vi "Create Message.vi"(8 "error in (no error)":errorcluster, 11 "Message Name":string) -> (0 "error out":errorcluster, 3 "Message out":refnum<class "Message.lvclass">)   [LabVIEW 2009, in "LapDog.Messaging.v2.lvlib" / "Message.lvclass"]
doc: "Creates a message object with the given name. If no name is wired to the input the message name is the same as the class name.\n\nThis method executes regardless of the error in state."
uses:
  Message.lvclass
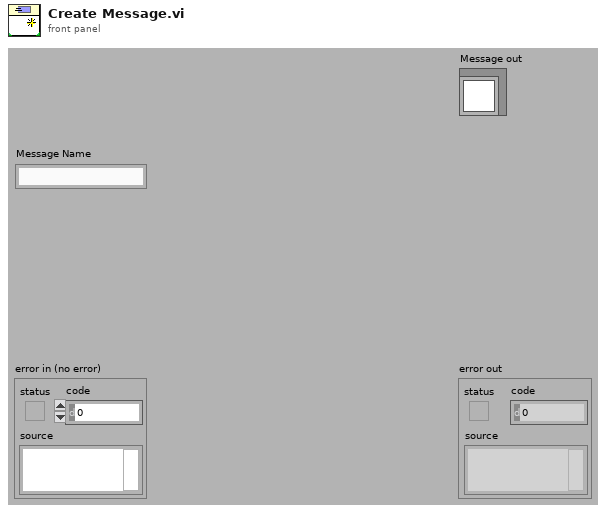
[diagram p1: front panel]
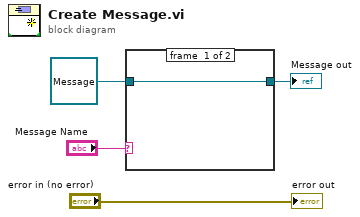
[diagram p0: block diagram]
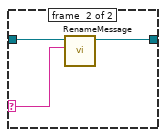
[diagram p2: hidden frame]
diagram:
  n1 = case shown="Default" "Message Name" {
    selector: "Message Name" -> [_ w6]
    tunnel: refnum<class "Message.lvclass"> refnum ("Message in") -> [w5 w8]
    tunnel: [w5 w7] -> w2
    frame #0 {
    }
    frame #1 {
      n2 = call "RenameMessage.vi"("Message Name"=w6, "Message in"=w8) -> ("Message out"=w7:refnum<class "Message.lvclass">)  [unwired: 8 in, 1 out]
    }
  }
  "Message out" <- w2
  "error out" <- "error in (no error)"
